vi "from_SGL.vi"(8 "error_in":errorcluster, 11 "I16":sgl) -> (0 "error_out":errorcluster, 3 "byte_array":u8[](array[numeric]))   [LabVIEW 2020]
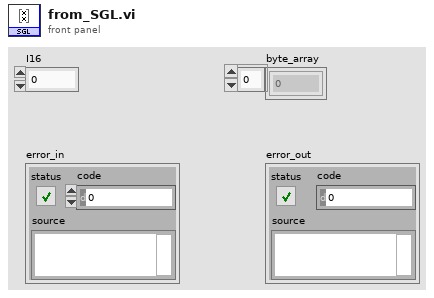
[diagram p1: front panel]
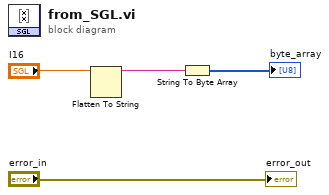
[diagram p0: block diagram]
diagram:
  n1 = Flatten To String(anything="I16") -> (data string=w2:string)  [unwired: 3 in, 2 out]
  n2 = String To Byte Array(string=w2) -> (unsigned byte array=→"byte_array":u8[])
  "error_out" <- "error_in"
